vi "Write speed.vi"(10 "speed":dbl, 11 "shooter in":refnum<class "shooter.lvclass">) -> (3 "shooter out":refnum<class "shooter.lvclass">)   [LabVIEW 2015, in "shooter.lvclass"]
uses:
  shooter.lvclass
  shooter.lvclass/shooter.ctl
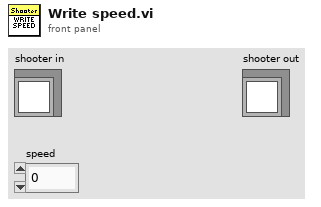
[diagram p1: front panel]
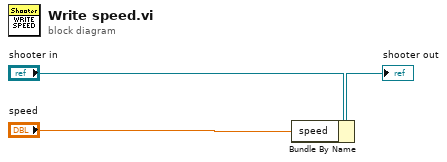
[diagram p0: block diagram]
diagram:
  n1 = Bundle By Name(cluster="shooter in", "speed"="speed") -> (→"shooter out":refnum<class "shooter.lvclass">)
